vi "n z out list.vi"(8 "error in (no error)":errorcluster, 10 "z":i16, 11 "n":u16) -> (0 "error out":errorcluster)   [LabVIEW 2015, in "SCANalone4x64.lvlib"]
doc: "__declspec(dllimport) void __stdcall n_z_out_list(unsigned short n, short z);"
uses:
  <userlib>/SCANalone4x64/SCANalone4x64.lvlib
  <userlib>/SCANalone4x64/SCANalone4x64.dll
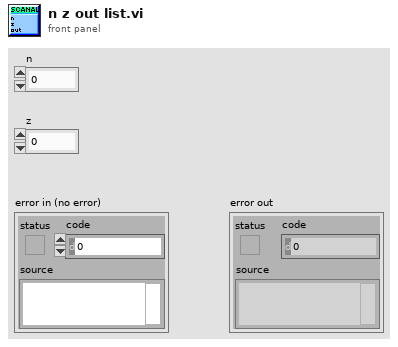
[diagram p1: front panel]
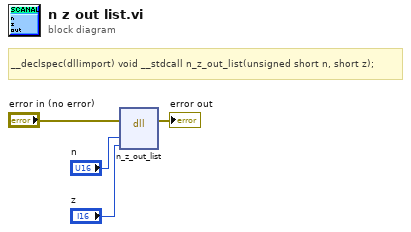
[diagram p0: block diagram]
diagram:
  # "__declspec(dllimport) void __stdcall n_z_out_list(unsigned short n, short z);"
  n1 = dll-call lib="C:/Program Files/National Instruments/LabVIEW 2015/user.lib/SCANalone4x64/SCANalone4x64.*" fn="n_z_out_list"(error in="error in (no error)", "n"="n", "z"="z") -> (error out=→"error out":errorcluster)  [unwired: 5 in, 1 out]
